vi "Create DAT Comments.vi"(8 "error in":errorcluster, 10 "Additional comments":string, 11 "Retrieve and Visualize":refnum<class "Retrieve and Visualize.lvclass">) -> (0 "error out":errorcluster, 3 "Retrieve and Visualize out":refnum<class "Retrieve and Visualize.lvclass">)   [LabVIEW 2020, in "Retrieve and Visualize.lvclass"]
uses:
  Retrieve and Visualize.lvclass
  Retrieve and Visualize.lvclass/Retrieve and Visualize.ctl
panel:
  out "IV setup":T1
  out "DAT Comments":string
  out "Field Period":i32
  out "# of fields/Tempertatures":i32
  out "Decimate point":dbl
  out "comments IN":string
  out "Scan names":string[](array[string])
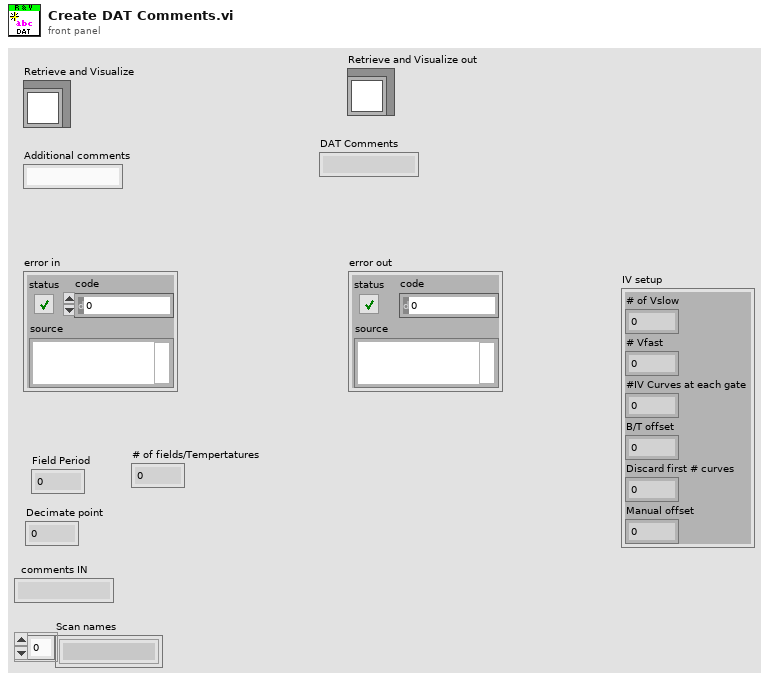
[diagram p1: front panel]
types:
  T1 = cluster{"# of Vslow":i32, "# Vfast":i32, "#IV Curves at each gate":i32, "B/T offset":i32, "Discard first # curves":i32, "Manual offset":i32}
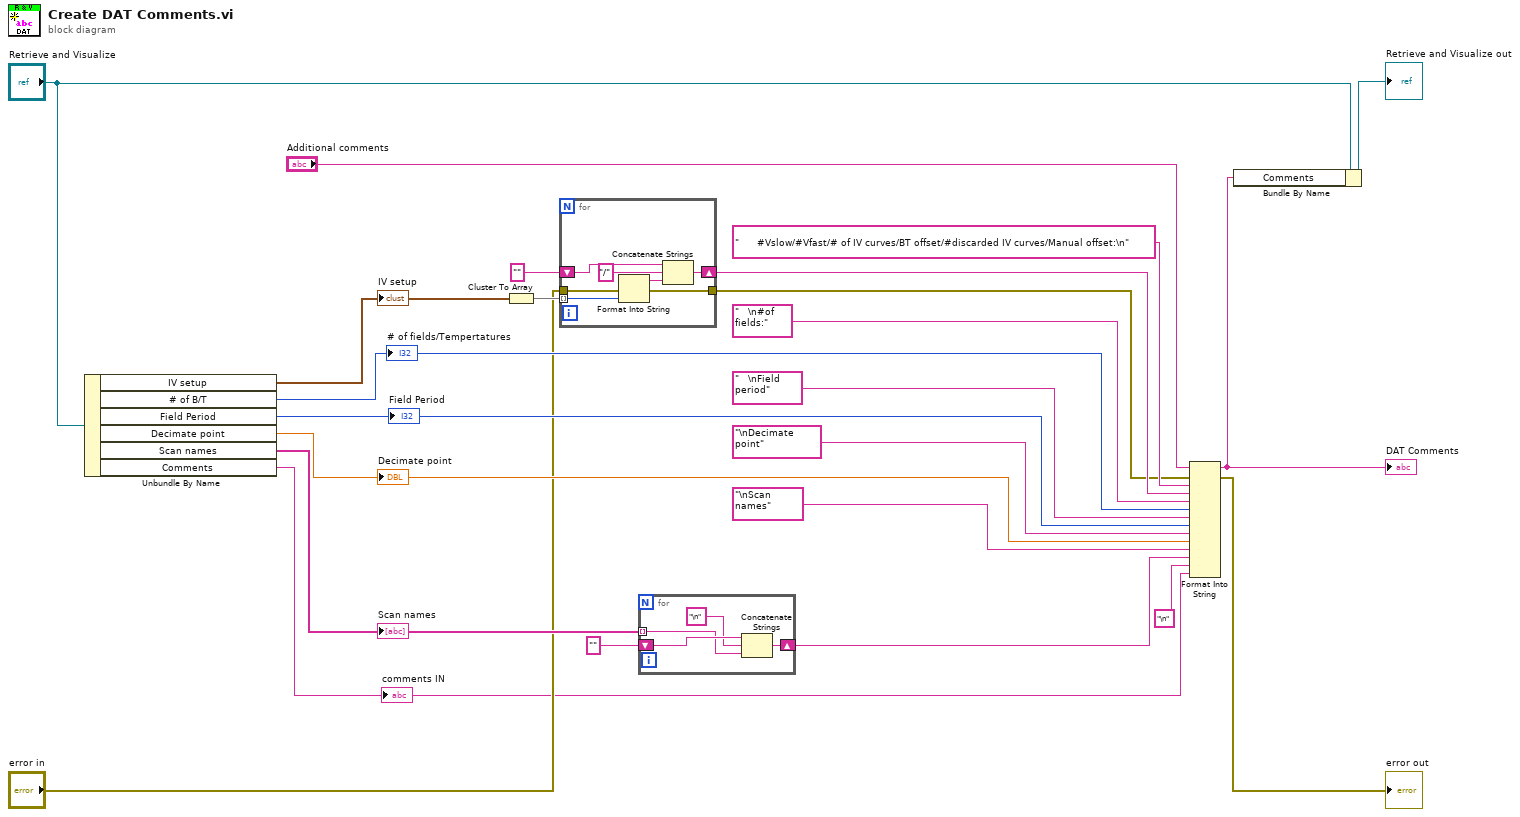
[diagram p0: block diagram]
diagram:
  n1 = Unbundle By Name("Retrieve and Visualize") -> ("IV setup"=w10:T1, "# of B/T"=w15:i32, "Field Period"=w14:i32, "Decimate point"=w13:dbl, "Scan names"=w12:string[], "Comments"=w1:string)
  "Scan names" <- w12
  "comments IN" <- w1
  "Decimate point" <- w13
  "# of fields/Tempertatures" <- w15
  "Field Period" <- w14
  "IV setup" <- w10
  n2 = Cluster To Array(cluster=w10) -> (array=w16:i32[])
  n3 = for {
    tunnel: w16 -> [w31] mode=indexing
    shift-right: [w28] -> w19
    shift-left: "" -> [w27]
    tunnel: "error in" -> [w26]
    tunnel: [w25] -> w3
    n4 = Format Into String(error in=w26, w31) -> (resulting string=w30:string, error out=w25:errorcluster)  [unwired: 2 in]
    n5 = Concatenate Strings(w27, "/" ("string"), w30) -> (w28:string)
  }
  n6 = for {
    tunnel: w12 -> [w33] mode=indexing
    shift-right: [w35] -> w23
    shift-left: "" -> [w34]
    n7 = Concatenate Strings(w34, "\n" ("string"), w33) -> (w35:string)
  }
  n8 = Format Into String(initial string="Additional comments", error in=w3, "      #Vslow/#Vfast/# of IV curves/BT offset/#discarded IV curves/Manual offset:\n" ("string"), w19, "   \n#of fields:" ("string"), w15, "   \nField period" ("string"), w14, "\nDecimate point", w13, "\nScan names", w23, "\n" ("input 11"), w1) -> (resulting string=w6:string, error out=→"error out":errorcluster)  [unwired: 1 in]
  "DAT Comments" <- w6
  n9 = Bundle By Name(cluster="Retrieve and Visualize", "Comments"=w6) -> (→"Retrieve and Visualize out":refnum<class "Retrieve and Visualize.lvclass">)
